vi "LD2018_ブロック崩し_Log取り.vi"(4 "方向 1":i32, 5 "方向 2":i32, 6 "BOTTOM":i16, 7 "time string":string, 8 "R":i16, 9 "TOP":i16, 10 "L":i16, 11 "file path (dialog if empty)":path) -> ()   [LabVIEW 2016]
uses:
  <vilib>/Utility/file.llb/Write Delimited Spreadsheet (string).vi
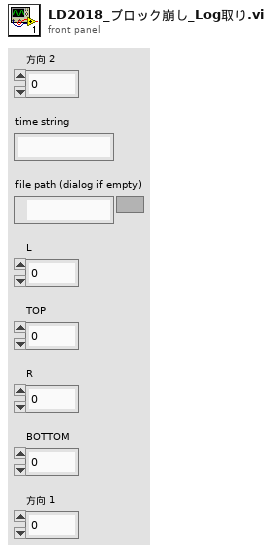
[diagram p1: front panel]
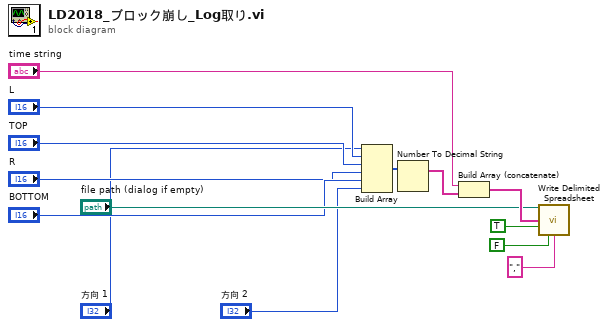
[diagram p0: block diagram]
diagram:
  n1 = Build Array("方向 1", "L", "TOP", "R", "BOTTOM", "方向 2") -> (w7:i32[])
  n2 = Number To Decimal String(number=w7) -> (decimal integer string=w12:string[])  [unwired: 1 in]
  n3 = Build Array (concatenate)("time string", w12) -> (w14:string[])
  n4 = call-poly <vilib>:"Write Delimited Spreadsheet.vi"("file path (dialog if empty)"="file path (dialog if empty)", "1D data"=w14, "append to file? (new file:F)"=TRUE, "transpose? (no:F)"=FALSE, "delimiter (\\t)"="," ("delimiter (\\t)")) -> ()  [unwired: 9 in, 2 out]
